vi "Sort Tree Items by Numerical order.vi"(6 "Reverse Order?":bool, 8 "error in":errorcluster, 9 "Sort Column":i32, 10 "Tag (\"\")":string, 11 "Data Tree":refnum<vi>) -> (0 "error out":errorcluster)   [LabVIEW 2013]
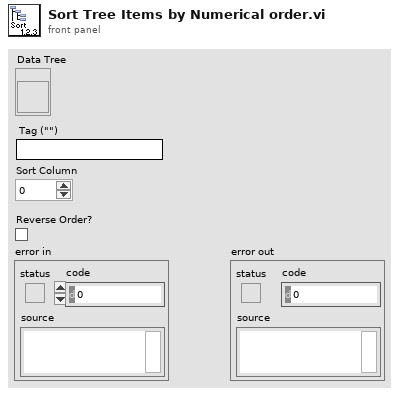
[diagram p1: front panel]
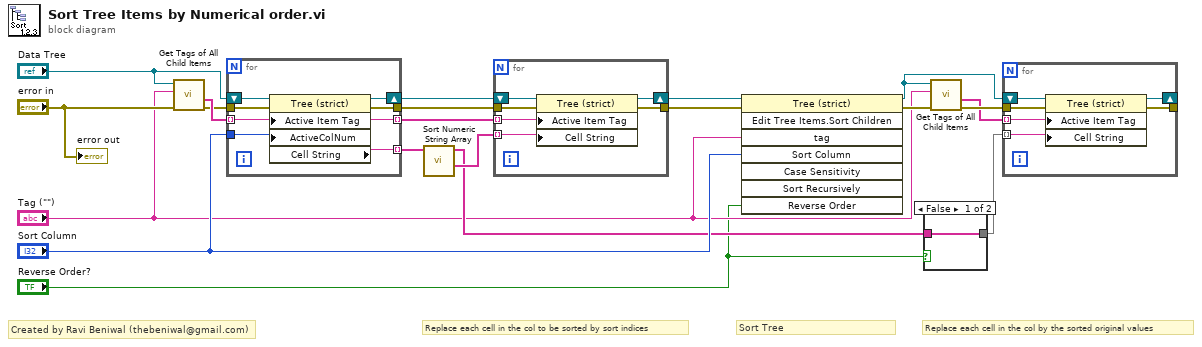
[diagram p0: block diagram]
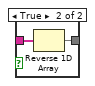
[diagram p2: hidden frame]
diagram:
  # "Replace each cell in the col by the sorted original values"
  # "Sort Tree"
  # "Created by Ravi Beniwal (thebeniwal@gmail.com)"
  # "Replace each cell in the col to be sorted by sort indices"
  n1 = call "Get Tags of All Child Items.vi"("error in"="error in", "Parent Tag"="Tag (\"\")", "Tree Ref in"="Data Tree") -> ("error out"=w17:errorcluster, "Tags of All Child Items"=w18:string[])  [unwired: 4 in, 3 out]
  n2 = for {
    tunnel: [w24] -> w11
    shift-right: [w23] -> w14
    shift-left: "Data Tree" -> [w27]
    tunnel: w18 -> [w21] mode=indexing
    tunnel: w17 -> [w26]
    tunnel: "Sort Column" -> [w25]
    tunnel: [w22] -> w15 mode=indexing
    tunnel: [w21] -> w12 mode=indexing
    n3 = property class="Tree (strict)"(reference=w27, error in=w26, "Active Item Tag"=w21, "ActiveColNum"=w25) -> (reference out=w23:refnum<vi>, error out=w24:errorcluster, "Cell String"=w22:string)
  }
  n4 = call "Sort Numeric String Array.vi"("Array Values"=w15) -> ("Column Values for Sorting as String"=w10:string[], "Sorted Array Values"=w8:string[])  [unwired: 9 in]
  n5 = for {
    tunnel: [w31] -> w9
    shift-right: [w30] -> w13
    shift-left: w14 -> [w33]
    tunnel: w12 -> [w28] mode=indexing
    tunnel: w11 -> [w32]
    tunnel: w10 -> [w29] mode=indexing
    n6 = property class="Tree (strict)"(reference=w33, error in=w32, "Active Item Tag"=w28, "Cell String"=w29) -> (reference out=w30:refnum<vi>, error out=w31:errorcluster)
  }
  n7 = invoke on="Invoke Node" class="Tree (strict)" method="Edit Tree Items.Sort Children"(reference=w13, error in=w9, "tag"="Tag (\"\")", "Sort Column"="Sort Column", "Reverse Order"="Reverse Order?") -> (reference out=w5:refnum<vi>, error out=w7:errorcluster)  [unwired: 3 in, 6 out]
  n8 = case shown="False" "Reverse Order?" {
    tunnel: w8 -> [w34 w36]
    tunnel: [w34 w35] -> w2
    frame False {
    }
    frame True {
      n9 = Reverse 1D Array(array=w36) -> (reversed array=w35:string[])
    }
  }
  n10 = call "Get Tags of All Child Items.vi"("error in"=w7, "Parent Tag"="Tag (\"\")", "Tree Ref in"=w5) -> ("error out"=w6:errorcluster, "Tags of All Child Items"=w3:string[])  [unwired: 4 in, 3 out]
  n11 = for {
    tunnel: [w39] -> _
    shift-right: [w38] -> _
    shift-left: w5 -> [w41]
    tunnel: w3 -> [w42] mode=indexing
    tunnel: w6 -> [w40]
    tunnel: w2 -> [w37] mode=indexing
    n12 = property class="Tree (strict)"(reference=w41, error in=w40, "Active Item Tag"=w42, "Cell String"=w37) -> (reference out=w38:refnum<vi>, error out=w39:errorcluster)
  }
  "error out" <- "error in"
